vi "Reef Align Play Path.vi"(4 "PID setpoint":dbl=-0.49, 6 "Tag ID":dbl=19.0, 7 "PID Constants":T1={"P Gain"=0.09, "I Gain"=0.0, "D Gain"=0.0, "F Gain"=0.08, "I Zone"=0.0, "Min Output"=-1.0, "Max Output"=1.0}, 8 "Operation":T2=enum."Reef Align", 9 "Auto Data":T14={"Auto Velocities"=[{"X Velocity"=-1.8462498434907955, "Y Velocity"=7.056933814139086, "Rotational \nVelocity"=-0.0}, {"X Velocity"=-1.991747061129249, "Y Velocity"=7.535671418858484, "Rotational \nVelocity"=-7.2}, {"X Velocity"=-2.1476402119148625, "Y Velocity"=8.011584634482254, "Rotational \nVelocity"=-10.052643775939941}, {"X Velocity"=-2.306896278662117, "Y Velocity"=8.486490625788083, "Rotational \nVelocity"=-10.052643775939941}, {"X Velocity"=-2.4695100913190724, "Y Velocity"=8.960371657345226, "Rotational \nVelocity"=-10.052643775939941}, {"X Velocity"=-2.635476396794092, "Y Velocity"=9.433210017677535, "Rotational \nVelocity"=-10.052643775939941}, {"X Velocity"=-2.6685615639393947, "Y Velocity"=9.423903981638178, "Rotational \nVelocity"=-10.052643775939941}, {"X Velocity"=-2.701613872254829, "Y Velocity"=9.414481906133277, "Rotational \nVelocity"=-10.052643775939941}, {"X Velocity"=-2.7346329147570203, "Y Velocity"=9.404943907179781, "Rotational \nVelocity"=-10.052643775939941}, {"X Velocity"=-2.6263332099505634, "Y Velocity"=8.91566678376851, "Rotational \nVelocity"=-10.052643775939941}, {"X Velocity"=-2.5146351435076726, "Y Velocity"=8.427271425386172, "Rotational \nVelocity"=-10.052643775939941}, {"X Velocity"=-2.3995435908884546, "Y Velocity"=7.939775651158667, "Rotational \nVelocity"=-10.052643775939941}, {"X Velocity"=-2.2810635107418573, "Y Velocity"=7.453197256780454, "Rotational \nVelocity"=-10.052643775939941}, {"X Velocity"=-2.1591999448009993, "Y Velocity"=6.967554014150215, "Rotational \nVelocity"=-10.052643775939941}, {"X Velocity"=-2.0339580177769934, "Y Velocity"=6.482863671006963, "Rotational \nVelocity"=-10.052643775939941}, {"X Velocity"=-1.9053429372511914, "Y Velocity"=5.99914395056661, "Rotational \nVelocity"=-10.052643775939941}, {"X Velocity"=-1.7733599935659488, "Y Velocity"=5.516412551158996, "Rotational \nVelocity"=-10.052643775939941}, {"X Velocity"=-1.63801455971383, "Y Velocity"=5.034687145865371, "Rotational \nVelocity"=-10.052643775939941}, {"X Velocity"=-1.4993120912253046, "Y Velocity"=4.553985382156366, "Rotational \nVelocity"=-10.052643775939941}, {"X Velocity"=-1.3572581260549188, "Y Velocity"=4.074324881530425, "Rotational \nVelocity"=-10.052643775939941}, {"X Velocity"=-1.2118582844659433, "Y Velocity"=3.595723239152738, "Rotational \nVelocity"=-10.052643775939941}, {"X Velocity"=-1.0631182689134988, "Y Velocity"=3.118198023494648, "Rotational \nVelocity"=-10.052643775939941}, {"X Velocity"=-0.9110438639261721, "Y Velocity"=2.641766775973572, "Rotational \nVelocity"=-10.052643775939941}, {"X Velocity"=-0.7556409359861169, "Y Velocity"=2.166447010593411, "Rotational \nVelocity"=-10.052643775939941}, {"X Velocity"=-0.5969154334076338, "Y Velocity"=1.692256213585474, "Rotational \nVelocity"=-10.052643775939941}, {"X Velocity"=-0.4348733862142511, "Y Velocity"=1.2192118430499221, "Rotational \nVelocity"=-10.052643775939941}, {"X Velocity"=-0.26947258503234844, "Y Velocity"=0.7473487535270189, "Rotational \nVelocity"=-9.867414283752396}, {"X Velocity"=-0.1001328097589842, "Y Velocity"=0.2768976473427397, "Rotational \nVelocity"=-2.6674142837523886}, {"X Velocity"=-0.0, "Y Velocity"=0.0, "Rotational \nVelocity"=-0.0}], "Auto Positions"=[{"x"=0.8100058273974486, "y"=-3.967975741983552, "th"=5.222202301025391}, {"x"=0.7603878706355013, "y"=-3.830783760791278, "th"=5.0782023010253905}, {"x"=0.7073688364180365, "y"=-3.68418791485404, "th"=4.877149425506592}, {"x"=0.6509487247450543, "y"=-3.5281882041718386, "th"=4.676096549987793}, {"x"=0.5911275356165546, "y"=-3.3627846287446737, "th"=4.475043674468994}, {"x"=0.5279052690325376, "y"=-3.1879771885725448, "th"=4.273990798950195}, {"x"=0.46128192499300325, "y"=-3.0037658836554524, "th"=4.072937923431397}, {"x"=0.39465858095346884, "y"=-2.8195545787383596, "th"=3.8718850479125977}, {"x"=0.32803523691393444, "y"=-2.6353432738212668, "th"=3.6708321723937987}, {"x"=0.26141189287440003, "y"=-2.451131968904174, "th"=3.469779296875}, {"x"=0.198189626290383, "y"=-2.276324528732045, "th"=3.2687264213562015}, {"x"=0.1383684371618834, "y"=-2.1109209533048796, "th"=3.0676735458374025}, {"x"=0.0819483254889012, "y"=-1.954921242622678, "th"=2.8666206703186035}, {"x"=0.02892929127143639, "y"=-1.8083253966854402, "th"=2.6655677947998044}, {"x"=-0.020688665490511016, "y"=-1.671133415493166, "th"=2.4645149192810054}, {"x"=-0.06690554479694102, "y"=-1.5433452990458556, "th"=2.2634620437622064}, {"x"=-0.10972134664785363, "y"=-1.4249610473435088, "th"=2.0624091682434074}, {"x"=-0.14913607104324883, "y"=-1.315980660386126, "th"=1.8613562927246083}, {"x"=-0.18514971798312663, "y"=-1.2164041381737067, "th"=1.6603034172058093}, {"x"=-0.21776228746748705, "y"=-1.1262314807062512, "th"=1.4592505416870103}, {"x"=-0.24697377949633004, "y"=-1.0454626879837594, "th"=1.2581976661682113}, {"x"=-0.27278419406965565, "y"=-0.9740977600062313, "th"=1.0571447906494127}, {"x"=-0.29519353118746383, "y"=-0.9121366967736668, "th"=0.8560919151306141}, {"x"=-0.31420179084975464, "y"=-0.8595794982860661, "th"=0.6550390396118155}, {"x"=-0.329808973056528, "y"=-0.816426164543429, "th"=0.45398616409301695}, {"x"=-0.342015077807784, "y"=-0.7826766955457557, "th"=0.2529332885742184}, {"x"=-0.35082010510352263, "y"=-0.7583310912930461, "th"=0.055585002899170455}, {"x"=-0.3562240549437438, "y"=-0.7433893517853002, "th"=0.002236717224122664}, {"x"=-0.35822692732844763, "y"=-0.737851477022518, "th"=0.002236717224122664}], "Auto Commands"=[], "Zero Velocity?"=[]}, 10 "Motors":T3={"Drive Motors (NEO)"={"Left Front"={"DeviceStatus"={"status"=FALSE, "code"=0, "source"=""}, "Type"=enum."CAN", "PWM"={"PWM Channel"=enum."Invalid", "DeadBand"={"Name"="", "maxPositivePwm"=0, "minPositivePwm"=0, "centerPwm"=0, "maxNegativePwm"=0, "minNegativePwm"=0, "angularRange"=0}}, "CAN"={"Device Number"=1, "SetOutput VI Ref"=variant(refnum<vi> refnum), "GetOutput VI Ref"=variant(refnum<vi> refnum), "Enable VI Ref"=variant(refnum<vi> refnum), "Disable VI Ref"=variant(refnum<vi> refnum), "Data"=variant(cluster{"Ext ID":u32, "CAN Timeout":u32, "Inverted No WPILib":bool, "Has Configured Limit Sw":bool, "Has Configured Alt Encoder":bool, "SPARK Model":enum16{"SPARK MAX", "SPARK Flex", "Unknown"}, "CAN Max Retries":u32, "CAN Timeout (ms)":u32, "Status 0 Period (ms)":u32, "Status 1 Period (ms)":u32, "Status 2 Period (ms)":u32, "Status 3 Period (ms)":u32, "Status 4 Period (ms)":u32, "Status 5 Period (ms)":u32, "Status 6 Period (ms)":u32, "Status 7 Period (ms)":u32, "Status Frame Timeout (ms)":u32} {"Ext ID"=33882113, "CAN Timeout"=0, "Inverted No WPILib"=FALSE, "Has Configured Limit Sw"=FALSE, "Has Configured Alt Encoder"=FALSE, "SPARK Model"=enum."SPARK Flex", "CAN Max Retries"=5, "CAN Timeout (ms)"=20, "Status 0 Period (ms)"=10, "Status 1 Period (ms)"=250, "Status 2 Period (ms)"=20, "Status 3 Period (ms)"=20, "Status 4 Period (ms)"=20, "Status 5 Period (ms)"=20, "Status 6 Period (ms)"=20, "Status 7 Period (ms)"=20, "Status Frame Timeout (ms)"=500})}, "Invert"=FALSE, "DIO PWM"={"PWM \"Enable\" Channel"=enum."Invalid", "DIOChannel"=enum."Invalid", "PWM Rate"=0.0}}, "Left Back"={"DeviceStatus"={"status"=FALSE, "code"=0, "source"=""}, "Type"=enum."CAN", "PWM"={"PWM Channel"=enum."Invalid", "DeadBand"={"Name"="", "maxPositivePwm"=0, "minPositivePwm"=0, "centerPwm"=0, "maxNegativePwm"=0, "minNegativePwm"=0, "angularRange"=0}}, "CAN"={"Device Number"=3, "SetOutput VI Ref"=variant(refnum<vi> refnum), "GetOutput VI Ref"=variant(refnum<vi> refnum), "Enable VI Ref"=variant(refnum<vi> refnum), "Disable VI Ref"=variant(refnum<vi> refnum), "Data"=variant(cluster{"Ext ID":u32, "CAN Timeout":u32, "Inverted No WPILib":bool, "Has Configured Limit Sw":bool, "Has Configured Alt Encoder":bool, "SPARK Model":enum16{"SPARK MAX", "SPARK Flex", "Unknown"}, "CAN Max Retries":u32, "CAN Timeout (ms)":u32, "Status 0 Period (ms)":u32, "Status 1 Period (ms)":u32, "Status 2 Period (ms)":u32, "Status 3 Period (ms)":u32, "Status 4 Period (ms)":u32, "Status 5 Period (ms)":u32, "Status 6 Period (ms)":u32, "Status 7 Period (ms)":u32, "Status Frame Timeout (ms)":u32} {"Ext ID"=33882115, "CAN Timeout"=0, "Inverted No WPILib"=FALSE, "Has Configured Limit Sw"=FALSE, "Has Configured Alt Encoder"=FALSE, "SPARK Model"=enum."SPARK Flex", "CAN Max Retries"=5, "CAN Timeout (ms)"=20, "Status 0 Period (ms)"=10, "Status 1 Period (ms)"=250, "Status 2 Period (ms)"=20, "Status 3 Period (ms)"=20, "Status 4 Period (ms)"=20, "Status 5 Period (ms)"=20, "Status 6 Period (ms)"=20, "Status 7 Period (ms)"=20, "Status Frame Timeout (ms)"=500})}, "Invert"=FALSE, "DIO PWM"={"PWM \"Enable\" Channel"=enum."Invalid", "DIOChannel"=enum."Invalid", "PWM Rate"=0.0}}, "Right Front"={"DeviceStatus"={"status"=FALSE, "code"=0, "source"=""}, "Type"=enum."CAN", "PWM"={"PWM Channel"=enum."Invalid", "DeadBand"={"Name"="", "maxPositivePwm"=0, "minPositivePwm"=0, "centerPwm"=0, "maxNegativePwm"=0, "minNegativePwm"=0, "angularRange"=0}}, "CAN"={"Device Number"=5, "SetOutput VI Ref"=variant(refnum<vi> refnum), "GetOutput VI Ref"=variant(refnum<vi> refnum), "Enable VI Ref"=variant(refnum<vi> refnum), "Disable VI Ref"=variant(refnum<vi> refnum), "Data"=variant(cluster{"Ext ID":u32, "CAN Timeout":u32, "Inverted No WPILib":bool, "Has Configured Limit Sw":bool, "Has Configured Alt Encoder":bool, "SPARK Model":enum16{"SPARK MAX", "SPARK Flex", "Unknown"}, "CAN Max Retries":u32, "CAN Timeout (ms)":u32, "Status 0 Period (ms)":u32, "Status 1 Period (ms)":u32, "Status 2 Period (ms)":u32, "Status 3 Period (ms)":u32, "Status 4 Period (ms)":u32, "Status 5 Period (ms)":u32, "Status 6 Period (ms)":u32, "Status 7 Period (ms)":u32, "Status Frame Timeout (ms)":u32} {"Ext ID"=33882117, "CAN Timeout"=0, "Inverted No WPILib"=FALSE, "Has Configured Limit Sw"=FALSE, "Has Configured Alt Encoder"=FALSE, "SPARK Model"=enum."SPARK Flex", "CAN Max Retries"=5, "CAN Timeout (ms)"=20, "Status 0 Period (ms)"=10, "Status 1 Period (ms)"=250, "Status 2 Period (ms)"=20, "Status 3 Period (ms)"=20, "Status 4 Period (ms)"=20, "Status 5 Period (ms)"=20, "Status 6 Period (ms)"=20, "Status 7 Period (ms)"=20, "Status Frame Timeout (ms)"=500})}, "Invert"=FALSE, "DIO PWM"={"PWM \"Enable\" Channel"=enum."Invalid", "DIOChannel"=enum."Invalid", "PWM Rate"=0.0}}, "Right Back"={"DeviceStatus"={"status"=FALSE, "code"=0, "source"=""}, "Type"=enum."CAN", "PWM"={"PWM Channel"=enum."Invalid", "DeadBand"={"Name"="", "maxPositivePwm"=0, "minPositivePwm"=0, "centerPwm"=0, "maxNegativePwm"=0, "minNegativePwm"=0, "angularRange"=0}}, "CAN"={"Device Number"=7, "SetOutput VI Ref"=variant(refnum<vi> refnum), "GetOutput VI Ref"=variant(refnum<vi> refnum), "Enable VI Ref"=variant(refnum<vi> refnum), "Disable VI Ref"=variant(refnum<vi> refnum), "Data"=variant(cluster{"Ext ID":u32, "CAN Timeout":u32, "Inverted No WPILib":bool, "Has Configured Limit Sw":bool, "Has Configured Alt Encoder":bool, "SPARK Model":enum16{"SPARK MAX", "SPARK Flex", "Unknown"}, "CAN Max Retries":u32, "CAN Timeout (ms)":u32, "Status 0 Period (ms)":u32, "Status 1 Period (ms)":u32, "Status 2 Period (ms)":u32, "Status 3 Period (ms)":u32, "Status 4 Period (ms)":u32, "Status 5 Period (ms)":u32, "Status 6 Period (ms)":u32, "Status 7 Period (ms)":u32, "Status Frame Timeout (ms)":u32} {"Ext ID"=33882119, "CAN Timeout"=0, "Inverted No WPILib"=FALSE, "Has Configured Limit Sw"=FALSE, "Has Configured Alt Encoder"=FALSE, "SPARK Model"=enum."SPARK Flex", "CAN Max Retries"=5, "CAN Timeout (ms)"=20, "Status 0 Period (ms)"=10, "Status 1 Period (ms)"=250, "Status 2 Period (ms)"=20, "Status 3 Period (ms)"=20, "Status 4 Period (ms)"=20, "Status 5 Period (ms)"=20, "Status 6 Period (ms)"=20, "Status 7 Period (ms)"=20, "Status Frame Timeout (ms)"=500})}, "Invert"=FALSE, "DIO PWM"={"PWM \"Enable\" Channel"=enum."Invalid", "DIOChannel"=enum."Invalid", "PWM Rate"=0.0}}}, "Steer Motors (NEO)"={"Left Front"={"DeviceStatus"={"status"=FALSE, "code"=0, "source"=""}, "Type"=enum."CAN", "PWM"={"PWM Channel"=enum."Invalid", "DeadBand"={"Name"="", "maxPositivePwm"=0, "minPositivePwm"=0, "centerPwm"=0, "maxNegativePwm"=0, "minNegativePwm"=0, "angularRange"=0}}, "CAN"={"Device Number"=2, "SetOutput VI Ref"=variant(refnum<vi> refnum), "GetOutput VI Ref"=variant(refnum<vi> refnum), "Enable VI Ref"=variant(refnum<vi> refnum), "Disable VI Ref"=variant(refnum<vi> refnum), "Data"=variant(cluster{"Ext ID":u32, "CAN Timeout":u32, "Inverted No WPILib":bool, "Has Configured Limit Sw":bool, "Has Configured Alt Encoder":bool, "SPARK Model":enum16{"SPARK MAX", "SPARK Flex", "Unknown"}, "CAN Max Retries":u32, "CAN Timeout (ms)":u32, "Status 0 Period (ms)":u32, "Status 1 Period (ms)":u32, "Status 2 Period (ms)":u32, "Status 3 Period (ms)":u32, "Status 4 Period (ms)":u32, "Status 5 Period (ms)":u32, "Status 6 Period (ms)":u32, "Status 7 Period (ms)":u32, "Status Frame Timeout (ms)":u32} {"Ext ID"=33882114, "CAN Timeout"=0, "Inverted No WPILib"=TRUE, "Has Configured Limit Sw"=FALSE, "Has Configured Alt Encoder"=FALSE, "SPARK Model"=enum."SPARK MAX", "CAN Max Retries"=5, "CAN Timeout (ms)"=20, "Status 0 Period (ms)"=10, "Status 1 Period (ms)"=250, "Status 2 Period (ms)"=20, "Status 3 Period (ms)"=20, "Status 4 Period (ms)"=20, "Status 5 Period (ms)"=20, "Status 6 Period (ms)"=20, "Status 7 Period (ms)"=20, "Status Frame Timeout (ms)"=500})}, "Invert"=FALSE, "DIO PWM"={"PWM \"Enable\" Channel"=enum."Invalid", "DIOChannel"=enum."Invalid", "PWM Rate"=0.0}}, "Left Back"={"DeviceStatus"={"status"=FALSE, "code"=0, "source"=""}, "Type"=enum."CAN", "PWM"={"PWM Channel"=enum."Invalid", "DeadBand"={"Name"="", "maxPositivePwm"=0, "minPositivePwm"=0, "centerPwm"=0, "maxNegativePwm"=0, "minNegativePwm"=0, "angularRange"=0}}, "CAN"={"Device Number"=4, "SetOutput VI Ref"=variant(refnum<vi> refnum), "GetOutput VI Ref"=variant(refnum<vi> refnum), "Enable VI Ref"=variant(refnum<vi> refnum), "Disable VI Ref"=variant(refnum<vi> refnum), "Data"=variant(cluster{"Ext ID":u32, "CAN Timeout":u32, "Inverted No WPILib":bool, "Has Configured Limit Sw":bool, "Has Configured Alt Encoder":bool, "SPARK Model":enum16{"SPARK MAX", "SPARK Flex", "Unknown"}, "CAN Max Retries":u32, "CAN Timeout (ms)":u32, "Status 0 Period (ms)":u32, "Status 1 Period (ms)":u32, "Status 2 Period (ms)":u32, "Status 3 Period (ms)":u32, "Status 4 Period (ms)":u32, "Status 5 Period (ms)":u32, "Status 6 Period (ms)":u32, "Status 7 Period (ms)":u32, "Status Frame Timeout (ms)":u32} {"Ext ID"=33882116, "CAN Timeout"=0, "Inverted No WPILib"=TRUE, "Has Configured Limit Sw"=FALSE, "Has Configured Alt Encoder"=FALSE, "SPARK Model"=enum."SPARK MAX", "CAN Max Retries"=5, "CAN Timeout (ms)"=20, "Status 0 Period (ms)"=10, "Status 1 Period (ms)"=250, "Status 2 Period (ms)"=20, "Status 3 Period (ms)"=20, "Status 4 Period (ms)"=20, "Status 5 Period (ms)"=20, "Status 6 Period (ms)"=20, "Status 7 Period (ms)"=20, "Status Frame Timeout (ms)"=500})}, "Invert"=FALSE, "DIO PWM"={"PWM \"Enable\" Channel"=enum."Invalid", "DIOChannel"=enum."Invalid", "PWM Rate"=0.0}}, "Right Front"={"DeviceStatus"={"status"=FALSE, "code"=0, "source"=""}, "Type"=enum."CAN", "PWM"={"PWM Channel"=enum."Invalid", "DeadBand"={"Name"="", "maxPositivePwm"=0, "minPositivePwm"=0, "centerPwm"=0, "maxNegativePwm"=0, "minNegativePwm"=0, "angularRange"=0}}, "CAN"={"Device Number"=6, "SetOutput VI Ref"=variant(refnum<vi> refnum), "GetOutput VI Ref"=variant(refnum<vi> refnum), "Enable VI Ref"=variant(refnum<vi> refnum), "Disable VI Ref"=variant(refnum<vi> refnum), "Data"=variant(cluster{"Ext ID":u32, "CAN Timeout":u32, "Inverted No WPILib":bool, "Has Configured Limit Sw":bool, "Has Configured Alt Encoder":bool, "SPARK Model":enum16{"SPARK MAX", "SPARK Flex", "Unknown"}, "CAN Max Retries":u32, "CAN Timeout (ms)":u32, "Status 0 Period (ms)":u32, "Status 1 Period (ms)":u32, "Status 2 Period (ms)":u32, "Status 3 Period (ms)":u32, "Status 4 Period (ms)":u32, "Status 5 Period (ms)":u32, "Status 6 Period (ms)":u32, "Status 7 Period (ms)":u32, "Status Frame Timeout (ms)":u32} {"Ext ID"=33882118, "CAN Timeout"=0, "Inverted No WPILib"=TRUE, "Has Configured Limit Sw"=FALSE, "Has Configured Alt Encoder"=FALSE, "SPARK Model"=enum."SPARK MAX", "CAN Max Retries"=5, "CAN Timeout (ms)"=20, "Status 0 Period (ms)"=10, "Status 1 Period (ms)"=250, "Status 2 Period (ms)"=20, "Status 3 Period (ms)"=20, "Status 4 Period (ms)"=20, "Status 5 Period (ms)"=20, "Status 6 Period (ms)"=20, "Status 7 Period (ms)"=20, "Status Frame Timeout (ms)"=500})}, "Invert"=FALSE, "DIO PWM"={"PWM \"Enable\" Channel"=enum."Invalid", "DIOChannel"=enum."Invalid", "PWM Rate"=0.0}}, "Right Back"={"DeviceStatus"={"status"=FALSE, "code"=0, "source"=""}, "Type"=enum."CAN", "PWM"={"PWM Channel"=enum."Invalid", "DeadBand"={"Name"="", "maxPositivePwm"=0, "minPositivePwm"=0, "centerPwm"=0, "maxNegativePwm"=0, "minNegativePwm"=0, "angularRange"=0}}, "CAN"={"Device Number"=8, "SetOutput VI Ref"=variant(refnum<vi> refnum), "GetOutput VI Ref"=variant(refnum<vi> refnum), "Enable VI Ref"=variant(refnum<vi> refnum), "Disable VI Ref"=variant(refnum<vi> refnum), "Data"=variant(cluster{"Ext ID":u32, "CAN Timeout":u32, "Inverted No WPILib":bool, "Has Configured Limit Sw":bool, "Has Configured Alt Encoder":bool, "SPARK Model":enum16{"SPARK MAX", "SPARK Flex", "Unknown"}, "CAN Max Retries":u32, "CAN Timeout (ms)":u32, "Status 0 Period (ms)":u32, "Status 1 Period (ms)":u32, "Status 2 Period (ms)":u32, "Status 3 Period (ms)":u32, "Status 4 Period (ms)":u32, "Status 5 Period (ms)":u32, "Status 6 Period (ms)":u32, "Status 7 Period (ms)":u32, "Status Frame Timeout (ms)":u32} {"Ext ID"=33882120, "CAN Timeout"=0, "Inverted No WPILib"=TRUE, "Has Configured Limit Sw"=FALSE, "Has Configured Alt Encoder"=FALSE, "SPARK Model"=enum."SPARK MAX", "CAN Max Retries"=5, "CAN Timeout (ms)"=20, "Status 0 Period (ms)"=10, "Status 1 Period (ms)"=250, "Status 2 Period (ms)"=20, "Status 3 Period (ms)"=20, "Status 4 Period (ms)"=20, "Status 5 Period (ms)"=20, "Status 6 Period (ms)"=20, "Status 7 Period (ms)"=20, "Status Frame Timeout (ms)"=500})}, "Invert"=FALSE, "DIO PWM"={"PWM \"Enable\" Channel"=enum."Invalid", "DIOChannel"=enum."Invalid", "PWM Rate"=0.0}}}, "Pigeon2"={"DeviceStatus"={"status"=FALSE, "code"=0, "source"=""}, "Device Number"=21, "Type"=352321536, "Device ID"=352321557, "Handle"=22044056, "UsageFrame"=0, "Library Path"=path "libCTRE_PhoenixCCI.so"}, "Radii (ft)"={"Left Front Position"=[-0.9375, 0.9375], "Left Back Position"=[-0.9375, -0.9375], "Right Front Position"=[0.9375, 0.9375], "Right Back Position"=[0.9375, -0.9375]}} {"Radii (ft)"."Right Back Position" format="%.2f"; "Radii (ft)"."Right Front Position" format="%.2f"; "Radii (ft)"."Left Back Position" format="%.2f"; "Radii (ft)"."Left Front Position" format="%.2f"; "Pigeon2"."Type" items=["CAN"=352321536, "TalonSRX"=33554432]}, 11 "AprilTag Offset":dbl=-60.0) -> (0 "Auto Done?":bool=TRUE)   [LabVIEW 2023]
uses:
  swerve/Type Definitions/Data/Robot Velocities.ctl
  swerve/Type Definitions/Hardware/Swerve Drives/(NEO-NEO-ThroughBore-Pigeon2) Swerve.ctl
  swerve/Type Definitions/Hardware/4 Motor Sets/(NEO & NEO 550) 4 Motor Set.ctl
  <vilib>/Rock Robotics/WPI/MotorControl/WPI_MotorControlDeviceRef.ctl
  <vilib>/Rock Robotics/WPI/MotorControl/WPI_MotorControlType.ctl
  <vilib>/Rock Robotics/SystemInterfaces/DIO/FPGA_DIOPWMChannel.ctl
  <vilib>/Rock Robotics/WPI/PWM/WPI_PWMDeadband.ctl
  <vilib>/Rock Robotics/SystemInterfaces/DIO/FPGA_DIOChannel.ctl
  <vilib>/Rock Robotics/WPI/ThirdParty/Phoenix-LabVIEW/Pigeon IMU/CTRE_PigeonIMU_DeviceRef.ctl
  <vilib>/Rock Robotics/WPI/ThirdParty/Phoenix-LabVIEW/Pigeon IMU/CTRE_PigeonIMU_ConnectionType.ctl
  swerve/Type Definitions/Data/Pod Positions.ctl
  Implementation/Drive Operations.ctl
  <vilib>/Platform/TimedLoop/XDataNode/timing_clust.ctl
  <vilib>/Platform/TimedLoop/XDataNode/nitl_modes.ctl
  <vilib>/Platform/TimedLoop/XDataNode/wakeup.ctl
  <vilib>/Rock Robotics/WPI/ThirdParty/REV Robotics/REVLib/Typedef/Spark MAX Control Type.ctl
  <vilib>/Rock Robotics/WPI/DriverStation/WPI_DriverStationRobotMode2.ctl
  c1434f1d-cc94-402a-bfa5-996335562ac8.vi
  <vilib>/Rock Robotics/Network Tables/NT Read Numeric Array.vi
  Framework/Robot Global Data.vi
  <vilib>/Platform/TimedLoop/XDataNode/XDataNode.xnode
  <vilib>/Platform/TimedLoop/XDataNode/XDNodeRunTimeDep.lvlib
panel:
  out "Delay":dbl=9.0
  in  "Forward Speed":dbl=3.0
  in  "forward time":i32=10
  in  "Aligned Threshold":dbl=25.0
  in  "Int per ft":dbl=0.75
  # "describes what the angle of the tag is (determined in Drive Controller)"
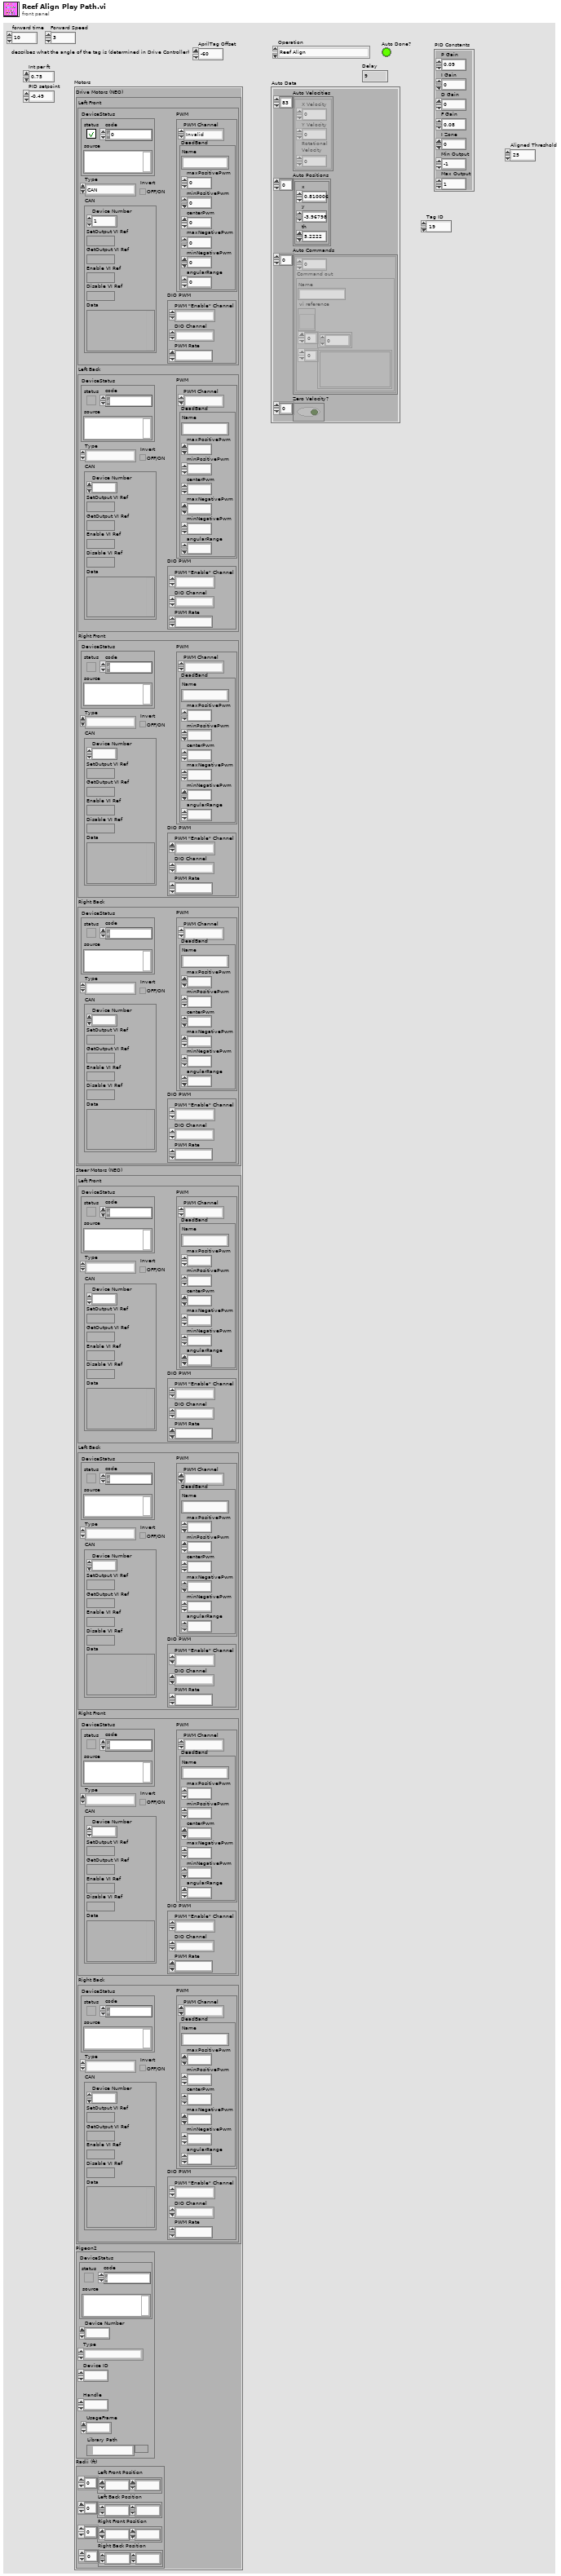
[diagram p1: front panel]
types:
  T1 = cluster{"P Gain":dbl, "I Gain":dbl, "D Gain":dbl, "F Gain":dbl, "I Zone":dbl, "Min Output":dbl, "Max Output":dbl}
  T2 = typedef "Drive Operations.ctl" = enum16{"Reserve", "Read Current", "Immediate", "Calibrate", "Reef Align", "Auto", "Old Reef Align"}
  T3 = typedef "(NEO-NEO-ThroughBore-Pigeon2) Swerve.ctl" = cluster{"Drive Motors (NEO)":T4, "Steer Motors (NEO)":T4, "Pigeon2":T10, "Radii (ft)":T12}
  T4 = typedef "(NEO & NEO 550) 4 Motor Set.ctl" = cluster{"Left Front":T5, "Left Back":T5, "Right Front":T5, "Right Back":T5}
  T5 = typedef "WPI_MotorControlDeviceRef.ctl" = cluster{"DeviceStatus":errorcluster, "Type":T6, "PWM":cluster{"PWM Channel":T7, "DeadBand":T8}, "CAN":cluster{"Device Number":u8, "SetOutput VI Ref":variant, "GetOutput VI Ref":variant, "Enable VI Ref":variant, "Disable VI Ref":variant, "Data":variant}, "Invert":bool, "DIO PWM":cluster{"PWM \"Enable\" Channel":T7, "DIOChannel":T9, "PWM Rate":dbl}}
  T6 = typedef "WPI_MotorControlType.ctl" = enum16{"PWM", "CAN", "DIO PWM"}
  T7 = typedef "FPGA_DIOPWMChannel.ctl" = enum8{"PWM 0", "PWM 1", "PWM 2", "PWM 3", "PWM 4", "PWM 5", "PWM 6", "PWM 7", "PWM 8", "PWM 9", "PWM MXP 0", "PWM MXP 1", "PWM MXP 2", "PWM MXP 3", "PWM MXP 4", "PWM MXP 5", "PWM MXP 6", "PWM MXP 7", "PWM MXP 8", "PWM MXP 9", "Invalid"}
  T8 = typedef "WPI_PWMDeadband.ctl" = cluster{"Name":string, "maxPositivePwm":i32, "minPositivePwm":i32, "centerPwm":i32, "maxNegativePwm":i32, "minNegativePwm":i32, "angularRange":u16}
  T9 = typedef "FPGA_DIOChannel.ctl" = enum8{"DIO 0", "DIO 1", "DIO 2", "DIO 3", "DIO 4", "DIO 5", "DIO 6", "DIO 7", "DIO 8", "DIO 9", "DIO MXP 0", "DIO MXP 1", "DIO MXP 2", "DIO MXP 3", "DIO MXP 4", "DIO MXP 5", "DIO MXP 6", "DIO MXP 7", "DIO MXP 8", "DIO MXP 9", "DIO MXP 10", "DIO MXP 11", "DIO MXP 12", "DIO MXP 13", "DIO MXP 14", "DIO MXP 15", "SPI Port CS1", "SPI Port CS2", "SPI Port CS3", "SPI Port MISO", "SPI Port MOSI", "Invalid"}
  T10 = typedef "CTRE_PigeonIMU_DeviceRef.ctl" = cluster{"DeviceStatus":errorcluster, "Device Number":u8, "Type":T11, "Device ID":u32, "Handle":u64, "UsageFrame":u32, "Library Path":path}
  T11 = typedef "CTRE_PigeonIMU_ConnectionType.ctl" = u32
  T12 = typedef "Pod Positions.ctl" = cluster{"Left Front Position":dbl[], "Left Back Position":dbl[], "Right Front Position":dbl[], "Right Back Position":dbl[]}
  T13 = typedef "Robot Velocities.ctl" = cluster{"X Velocity":dbl, "Y Velocity":dbl, "Rotational \nVelocity":dbl}
  T14 = cluster{"Auto Velocities":T13[], "Auto Positions":cluster{"x":dbl, "y":dbl, "th":dbl}[], "Auto Commands":cluster{dbl, "Command out":cluster{"Name":string, "vi reference":refnum<vi>, i32[], variant[]}}[], "Zero Velocity?":bool[]}
  T15 = cluster{"Time (s)":dbl, "Command out":cluster{"Name":string, "vi reference":refnum<vi>, i32[], variant[]}}
  T16 = typedef "Spark MAX Control Type.ctl" = enum16{"Percent VBus", "Voltage", "Velocity", "Position", "Smart Motion", "Current", "Smart Velocity", "MAXMotion Position", "MAXMotion Velocity"}
  T17 = cluster{"Left Front":dbl, "Left Back":dbl, "Right Front":dbl, "Right Back":dbl}
  T18 = typedef "XDNodeRunTimeDep.lvlib/timing_clust.ctl" = cluster{"Expected End [f-1]":u64, "Actual End [f-1]":u64, "Finished Late? [f-1]":bool, "Expected End [i-1]":u64, "Actual End [i-1]":u64, "Finished Late? [i-1]":bool, "Expected Start [i]":u64, "Actual Start [i]":u64, "Expected Start [f]":u64, "Actual Start [f]":u64, "Source Name":string, "Structure Name":string, "Period":i64, "Deadline":i64, "Offset":i64, "Start":i64, "Priority":i32, "Timeout":i32, "Mode":T19, "Wakeup Reason":T20, "Error":errorcluster, "Source Type":string, "Secondary Source Type":string, "Global End Time":u64, "Global Start Time":u64, "Frame Duration":u64, "Iteration Duration":u64, "Assigned CPU":i32, "I/O Scan Engine Mode":u32}
  T19 = typedef "XDNodeRunTimeDep.lvlib/nitl_modes.ctl" = enum32{"No Change", "Process missed periods, maintain original phase", "Discard missed periods, maintain original phase", "Process missed periods, ignore original phase", "Discard missed periods, ignore original phase"}
  T20 = typedef "XDNodeRunTimeDep.lvlib/wakeup.ctl" = enum32{"Normal", "Aborted", "Asynchronous wakeup", "Timing source error", "Timed loop error", "Timeout"}
  T21 = cluster{dbl, "Command out":cluster{"Name":string, "vi reference":refnum<vi>, i32[], variant[]}}[]
  T22 = cluster{"Field Centric":bool, "Reef Centric":bool}
  T23 = typedef "WPI_DriverStationRobotMode2.ctl" = enum16{"Autonomous Disabled", "Autonomous Enabled", "Teleop Disabled", "Teleop Enabled", "Disconnected", "Finish", "Test Disabled", "Test Enabled", "Emergency Stopped"}
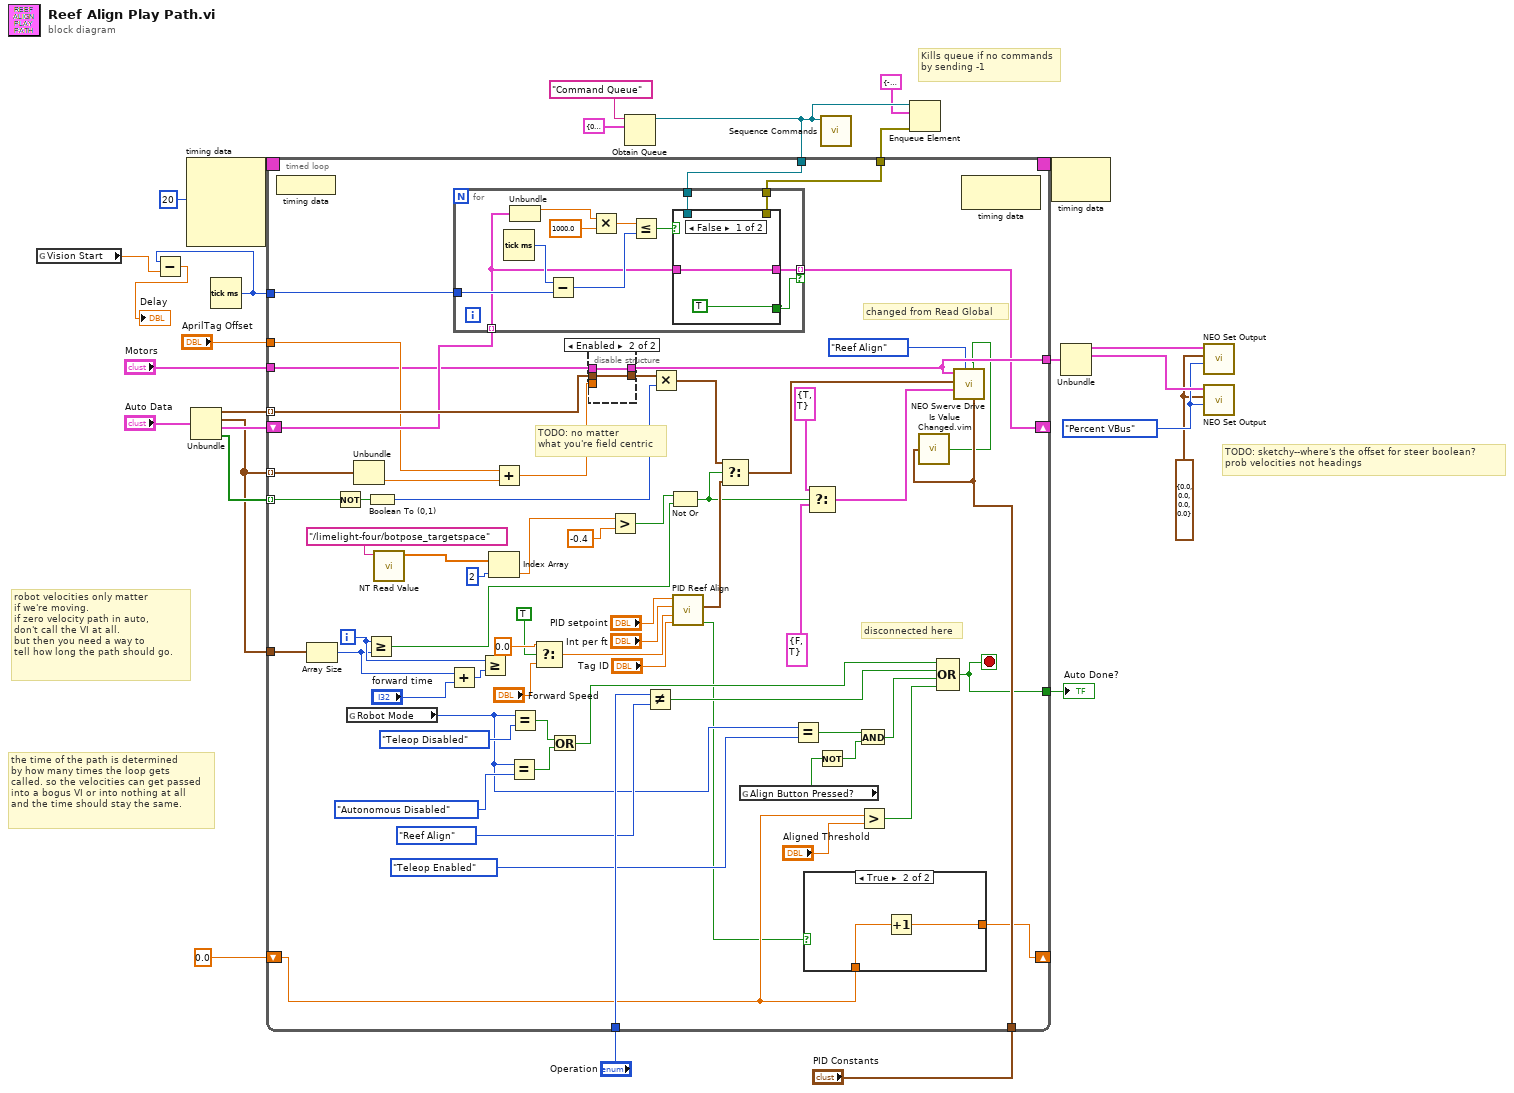
[diagram p0: block diagram]
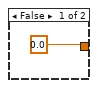
[diagram p2: hidden frame]
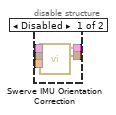
[diagram p3: hidden frame]
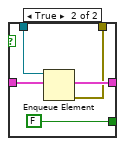
[diagram p4: hidden frame]
diagram:
  w13 = Spark_MAX_Control_Type."Percent VBus" ("Control Mode")
  w12 = T17 {"Left Front"=0.0, "Left Back"=0.0, "Right Front"=0.0, "Right Back"=0.0} ("Setpoints")
  # "the time of the path is determined\nby how many times the loop gets\ncalled. so the velocities can get passed\ninto a bogus VI or into nothing at all\nand the time should stay the same."
  # "robot velocities only matter\nif we're moving.\nif zero velocity path in auto,\ndon't call the VI at all.\nbut then you need a way to \ntell how long the path should go."
  # "TODO: sketchy--where's the offset for steer boolean?\nprob velocities not headings"
  # "Kills queue if no commands by sending -1"
  n1 = global read "Robot Global Data.vi" "Vision Start"() -> (w2:dbl)
  n2 = node-c288(i64 20 ("Period")) -> (w27:T18)  [unwired: 3 in]
  n3 = Unbundle("Auto Data") -> ("Auto Velocities"=w21:T13[], "Auto Positions"=w22:cluster{"x":dbl, "y":dbl, "th":dbl}[], "Auto Commands"=w23:T21, "Zero Velocity?"=w24:bool[])
  n4 = Tick Count (ms)() -> (millisecond timer value=w3:u32)
  n5 = Subtract(x=w3, y=w2) -> (x-y=→"Delay":dbl)
  n6 = Obtain Queue(name (unnamed)="Command Queue", element data type=T15 {"Time (s)"=0.0, "Command out"={"Name"="", "vi reference"=refnum, [], []}} ("element")) -> (queue out=w9:refnum<queue>)  [unwired: 3 in, 2 out]
  n7 = timed-loop {
    timing: w27 -> [_]
    timing-out: [_] -> w26
    tunnel: "Motors" -> [w49]
    tunnel: [w92] -> w11
    tunnel: w21 -> [w91] mode=indexing
    tunnel: w22 -> [w90] mode=indexing
    tunnel: w22 -> [w59]
    tunnel: w3 -> [w89]
    tunnel: w9 -> [w88]
    shift-right: [w86] -> _
    shift-left: w23 -> [w85]
    tunnel: w24 -> [w81] mode=indexing
    tunnel: [w73] -> w25
    tunnel: "Operation" -> [w80]
    tunnel: [w79] -> w8
    tunnel: "PID Constants" -> [w77]
    tunnel: "AprilTag Offset" -> [w72]
    shift-right: [w48] -> _
    shift-left: 0.0 -> [w47]
    i -> [w43]
    stop <- w73 stop-if-true
    # "TODO: no matter\nwhat you're field centric"
    # "changed from Read Global"
    # "disconnected here"
    n8 = node-c288() -> ()  [unwired: 1 in]
    n9 = Array Size(array=w59) -> (size(s)=w38:i32)
    n10 = Not(x=w81) -> (.not. x?=w84:bool)
    n11 = global read "Robot Global Data.vi" "Robot Mode"() -> (w64:T23)
    n12 = Unbundle(w90) -> ("th"=w70:dbl)  [unwired: 2 out]
    n13 = Greater Or Equal?(x=w43, y=w38) -> (x >= y?=w29:bool)
    n14 = Boolean To (0,1)(Boolean=w84) -> (0, 1=w83:i16)
    n15 = call-poly <vilib>:"NT Read Value.vi"("name"="/limelight-four/botpose_targetspace") -> ("value"=w34:dbl[])  [unwired: 8 in, 2 out]
    n16 = Add(x=w38, y="forward time") -> (x+y=w42:i32)
    n17 = for {
      tunnel: w89 -> [w113]
      tunnel: w88 -> [w107]
      tunnel: w85 -> [w104] mode=indexing
      tunnel: [w106] -> w86 mode=indexing if=w105
      tunnel: [w103] -> w79
      n18 = Tick Count (ms)() -> (millisecond timer value=w114:u32)
      n19 = Unbundle(w104) -> (w112:dbl)  [unwired: 1 out]
      n20 = Subtract(x=w114, y=w113) -> (x-y=w109:u32)
      n21 = Multiply(x=w112, y=1000.0) -> (x*y=w110:dbl)
      n22 = Less Or Equal?(x=w110, y=w109) -> (x <= y?=w108:bool)
      n23 = case shown="False" w108 {
        tunnel: w107 -> [_ w120]
        tunnel: w104 -> [w115 w119]
        tunnel: [w115 w119] -> w106
        tunnel: [TRUE FALSE] -> w105
        tunnel: [_ w117] -> w103
        frame False {
        }
        frame True {
          n24 = Enqueue Element(queue=w120, element=w119) -> (error out=w117:errorcluster)  [unwired: 2 in, 2 out]
        }
      }
    }
    n25 = Greater Or Equal?(x=w43, y=w42) -> ()  [unwired: 1 out]
    n26 = Index Array(array=w34, index=2) -> (element=w32:dbl)
    n27 = Add(x=w72, y=w70) -> (x+y=w71:dbl)
    n28 = Equal?(x=w64, y=WPI_DriverStationRobotMode2."Autonomous Disabled") -> (x = y?=w68:bool)
    n29 = Equal?(x=w64, y=WPI_DriverStationRobotMode2."Teleop Disabled") -> (x = y?=w67:bool)
    n30 = Select(t=0.0, s=TRUE, f="Forward Speed") -> (s? t:f=w44:dbl)
    n31 = Or(x=w67, y=w68) -> (x .or. y?=w66:bool)
    n32 = disable-structure shown="Enabled" {
      disable-tunnel: [w100 w102] -> w92
      disable-tunnel: w91 -> [w99 w101]
      disable-tunnel: w49 -> [w98 w102]
      disable-tunnel: [w97 w101] -> w78
      disable-tunnel: w71 -> [w96 _]
      frame Disabled {
        n33 = call "Swerve IMU Orientation Correction.vi"("Setpoint"=w96, "Robot Velocities In"=w99, "Motors In"=w98) -> ("Robot Velocities Out"=w97:T13, "Motors Out"=w100:T3)  [unwired: 7 in]
      }
      frame Enabled {
      }
    }
    n34 = Greater?(x=w32, y=-0.4) -> (0:w30:bool)
    n35 = Not Equal?(x=w80, y=Drive_Operations."Reef Align") -> (x != y?=w82:bool)
    n36 = Multiply(x=w78, y=w83) -> (x*y=w57:T13)
    n37 = Not Or(1:w29, 2:w30) -> (0:w31:bool)
    n38 = call "PID Reef Align.vi"("Tag ID"="Tag ID", "Y movement"=w44, "Int per ft"="Int per ft", "setpoint"="PID setpoint") -> ("PID Happy?"=w37:bool, "Robot Velocities Out"=w56:cluster{"output":dbl, "y":dbl, "y":dbl})  [unwired: 4 in]
    n39 = Select(t=w57, s=w31, f=w56) -> (s? t:f=w58:T13)
    n40 = global read "Robot Global Data.vi" "Align Button Pressed?"() -> (w69:bool)
    n41 = Equal?(x=w64, y=WPI_DriverStationRobotMode2."Teleop Enabled") -> (x = y?=w62:bool)
    n42 = case shown="True" w37 {
      tunnel: w47 -> [_ w95]
      tunnel: [0.0 w94] -> w48
      frame False {
      }
      frame True {
        n43 = Increment(x=w95) -> (x+1=w94:dbl)
      }
    }
    n44 = Select(t=T22 {"Field Centric"=TRUE, "Reef Centric"=TRUE} ("Drive Conditions"), s=w31, f=T22 {"Field Centric"=FALSE, "Reef Centric"=TRUE}) -> (s? t:f=w50:T22)
    n45 = Not(x=w69) -> (.not. x?=w61:bool)
    n46 = And(x=w62, y=w61) -> (x .and. y?=w60:bool)
    n47 = Greater?(x=w47, y="Aligned Threshold") -> (0:w45:bool)
    n48 = call "Is Value Changed.vim"("value"=w77) -> ("changed or first call?"=w76:bool)
    n49 = Compound Arithmetic op=OR(w66, w82, w60, w45) -> (w73:bool)
    n50 = call "NEO Swerve Drive.vi"("PID Constants"=w77, "Configure?"=w76, "Operation"=Drive_Operations."Reef Align", "Drive Conditions"=w50, "Robot Velocities"=w58, "Swerve Drive"=w92) -> ()  [unwired: 5 in, 1 out]
    n51 = node-c288() -> ()  [unwired: 1 in, 1 out]
  }
  "Auto Done?" <- w25
  n52 = call "Sequence Commands.vi"("queue in"=w9) -> ()  [unwired: 11 in]
  n53 = Enqueue Element(queue=w9, element=T15 {"Time (s)"=-1.0, "Command out"={"Name"="", "vi reference"=refnum, [], []}}, error in (no error)=w8) -> ()  [unwired: 1 in, 3 out]
  n54 = node-c288(w26) -> ()  [unwired: 1 out]
  n55 = Unbundle(w11) -> ("Drive Motors (NEO)"=w15:T4, "Steer Motors (NEO)"=w14:T4)  [unwired: 2 out]
  n56 = call "NEO Set Output.vi"("Control Mode"=w13, "Setpoints"=w12, "Motors"=w15) -> ()  [unwired: 9 in]
  n57 = call "NEO Set Output.vi"("Control Mode"=w13, "Setpoints"=w12, "Motors"=w14) -> ()  [unwired: 9 in]
